vi "DirecTemp.vi"(2 "error in (no error)":errorcluster, 3 "write buffer":string="2", 4 "baud rate (9600)":u32=38400, 5 "VISA resource name":refnum<visa-resource-name>) -> (0 "error out":errorcluster, 1 "read buffer":string)   [LabVIEW 2018]
uses:
  <vilib>/Instr/_visa.llb/VISA Configure Serial Port (Instr).vi
panel:
  out "return count":u32
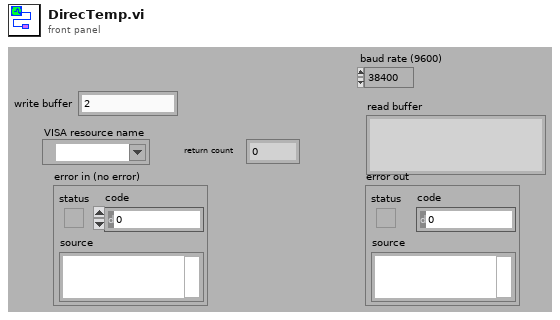
[diagram p1: front panel]
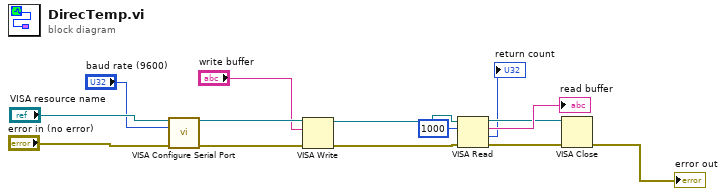
[diagram p0: block diagram]
diagram:
  n1 = call-poly "VISA Configure Serial Port"("VISA resource name"="VISA resource name", "baud rate (9600)"="baud rate (9600)", "error in (no error)"="error in (no error)") -> ("VISA resource name out"=w8:refnum<visa-resource-name>, "error out"=w7:errorcluster)  [unwired: 11 in]
  n2 = VISA Write(VISA resource name=w8, write buffer="write buffer", error in (no error)=w7) -> (VISA resource name out=w5:refnum<visa-resource-name>, error out=w4:errorcluster)  [unwired: 1 out]
  n3 = VISA Read(VISA resource name=w5, byte count=u32 1000, error in (no error)=w4) -> (VISA resource name out=w12:refnum<visa-resource-name>, read buffer=→"read buffer":string, return count=→"return count":u32, error out=w13:errorcluster)
  n4 = VISA Close(VISA resource name=w12, error in (no error)=w13) -> (error out=→"error out":errorcluster)
